vi "Shift Keys.vi"(10 "Upper / Lower Case":enum16{"Uppercase", "Lowercase"}(ring)=enum."Lowercase", 11 "Button Refs":T1) -> ()   [LabVIEW 2025]
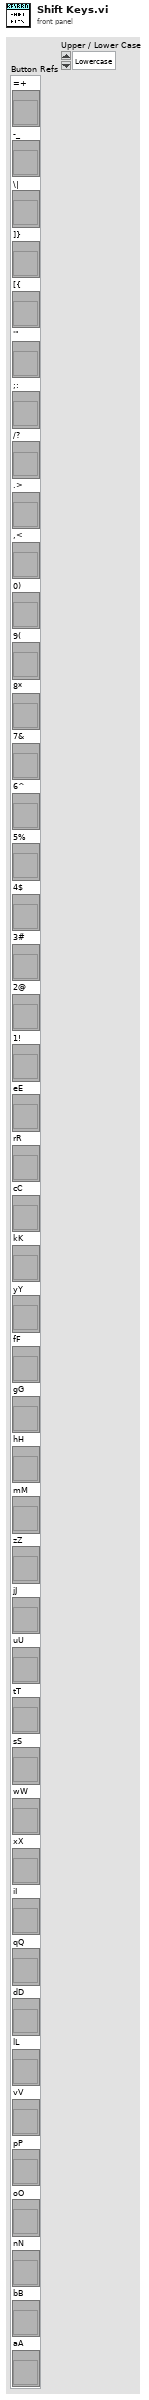
[diagram p1: front panel]
types:
  T1 = cluster{"=+":refnum<vi>, "-_":refnum<vi>, "\\|":refnum<vi>, "]}":refnum<vi>, "[{":refnum<vi>, "'\"":refnum<vi>, ";:":refnum<vi>, "/?":refnum<vi>, ".>":refnum<vi>, ",<":refnum<vi>, "0)":refnum<vi>, "9(":refnum<vi>, "8*":refnum<vi>, "7&":refnum<vi>, "6^":refnum<vi>, "5%":refnum<vi>, "4$":refnum<vi>, "3#":refnum<vi>, "2@":refnum<vi>, "1!":refnum<vi>, "eE":refnum<vi>, "rR":refnum<vi>, "cC":refnum<vi>, "kK":refnum<vi>, "yY":refnum<vi>, "fF":refnum<vi>, "gG":refnum<vi>, "hH":refnum<vi>, "mM":refnum<vi>, "zZ":refnum<vi>, "jJ":refnum<vi>, "uU":refnum<vi>, "tT":refnum<vi>, "sS":refnum<vi>, "wW":refnum<vi>, "xX":refnum<vi>, "iI":refnum<vi>, "qQ":refnum<vi>, "dD":refnum<vi>, "lL":refnum<vi>, "vV":refnum<vi>, "pP":refnum<vi>, "oO":refnum<vi>, "nN":refnum<vi>, "bB":refnum<vi>, "aA":refnum<vi>}
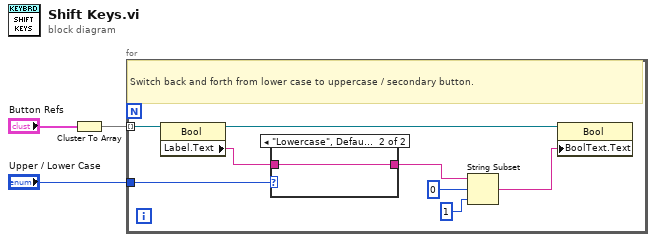
[diagram p0: block diagram]
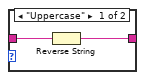
[diagram p2: hidden frame]
diagram:
  n1 = Cluster To Array(cluster="Button Refs") -> (array=w3:refnum<vi>[])
  n2 = for {
    tunnel: w3 -> [w11] mode=indexing
    tunnel: "Upper / Lower Case" -> [w4]
    # "Switch back and forth from lower case to uppercase / secondary button."
    n3 = property class="Bool"(reference=w11) -> (reference out=w9:refnum<vi>, "Label.Text"=w10:string)  [unwired: 1 in, 1 out]
    n4 = case shown="\"Lowercase\", Default" w4 {
      tunnel: w10 -> [w13 w14]
      tunnel: [w12 w14] -> w8
      frame "Uppercase" {
        n5 = Reverse String(1:w13) -> (0:w12:string)
      }
      frame "Lowercase", Default {
      }
    }
    n6 = String Subset(string=w8, offset (0)=0, length (rest)=1 ("length (rest)")) -> (substring=w6:string)
    n7 = property class="Bool"(reference=w9, "BoolText.Text"=w6) -> ()  [unwired: 1 in, 2 out]
  }
